vi "write dvr and enqueue.vi"(10 "Byte array":u8[](array[numeric]), 11 "Template in":refnum<class "Template.lvclass">) -> (0 "error out":errorcluster)   [LabVIEW 2020, in "Template.lvlib" / "Template.lvclass"]
doc: "Writes or creates the packets DVRs and enqueues them on the actor's queues."
uses:
  Template.lvclass
  Template.lvclass/Template.ctl
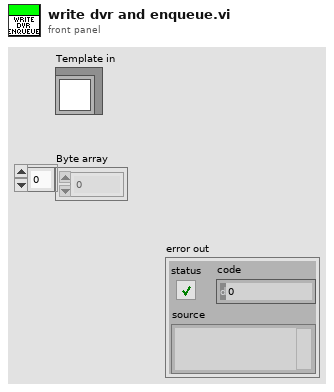
[diagram p1: front panel]
types:
  T1 = typedef "Template.lvlib/Template.lvclass/base actor queues.ctl" = cluster{"DVR Pool":refnum<queue>, "Actor's Data":refnum<queue>}
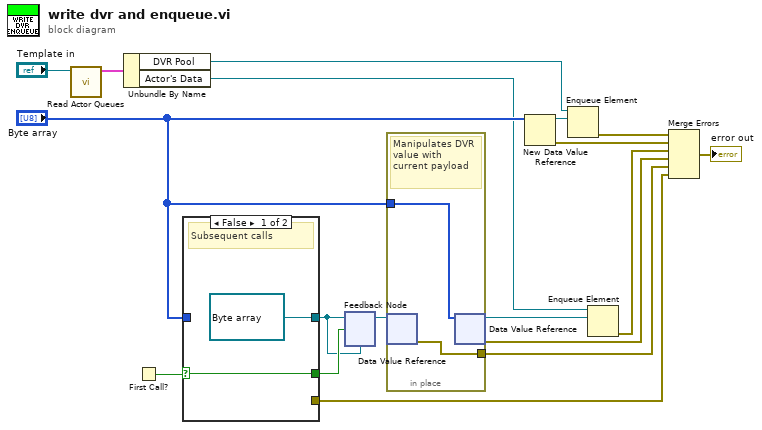
[diagram p0: block diagram]
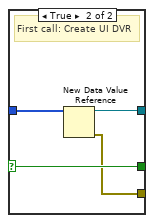
[diagram p2: hidden frame]
diagram:
  n1 = call "Read Actor Queues.vi"("Template in"="Template in") -> ("Base Actor Queues"=w1:T1)  [unwired: 10 in]
  n2 = Unbundle By Name(w1) -> ("DVR Pool"=w2:refnum<queue>, "Actor's Data"=w9:refnum<queue>)
  n3 = First Call?() -> (First Call?: T/F=w8:bool)
  n4 = case shown="False" w8 {
    selector: w8 -> [w20 w22]
    tunnel: "Byte array" -> [_ w24]
    tunnel: [refnum<data-value> refnum ("data value reference") w23] -> w11
    tunnel: [w20 w22] -> w13
    tunnel: [_ w21] -> w12
    frame False {
      # "Subsequent calls"
    }
    frame True {
      # "First call: Create UI DVR"
      n5 = New Data Value Reference(data value=w24) -> (data value reference=w23:refnum<data-value>, error out=w21:errorcluster)  [unwired: 1 in]
    }
  }
  n6 = feedback #1(w11) -> (w14:refnum<data-value>)
  n7 = feedback-in #1(w11, w13) -> ()
  n8 = in-place {
    in-place-border: "Byte array" -> [w26]
    in-place-border: [w25] -> w18
    # "Manipulates DVR value with current payload"
    n9 = in-place-dvr #2(w14) -> (w25:errorcluster)  [unwired: 1 out]
    n10 = in-place-dvr #2(w26) -> (w16:refnum<data-value>, w17:errorcluster)
  }
  n11 = New Data Value Reference(data value="Byte array") -> (data value reference=w3:refnum<data-value>, error out=w4:errorcluster)  [unwired: 1 in]
  n12 = Enqueue Element(queue=w2, element=w3) -> (error out=w7:errorcluster)  [unwired: 2 in, 2 out]
  n13 = Enqueue Element(queue=w9, element=w16) -> (error out=w10:errorcluster)  [unwired: 2 in, 2 out]
  n14 = Merge Errors(w7, w4, w10, w17, w18, w12) -> (→"error out":errorcluster)
